vi "Linux ip route get.vi"(8 "error in (no error)":errorcluster, 11 "address":refnum<class "IPv4 Network Address.lvclass">) -> (0 "error out":errorcluster, 3 "ip route get stdout":string, 5 "ip route get stderr":string)   [LabVIEW 2020, in "NI_WFCN.lvlib" / "IPv4 Network Address.lvclass"]
doc: "Linux: call `ip route get $ip` to determine if the specified address is routable."
uses:
  <vilib>/net/WFCN/Addressing/IPv4 Network Address/IPv4 Network Address.lvclass
  <vilib>/net/WFCN/NI_WFCN.lvlib
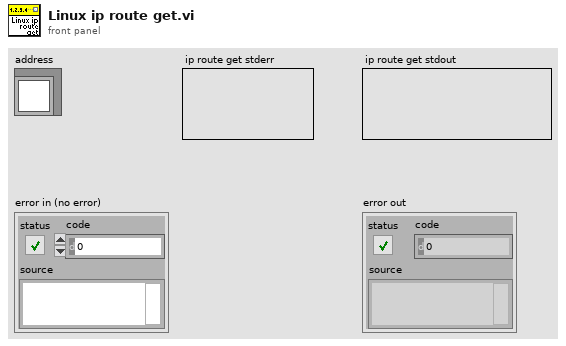
[diagram p1: front panel]
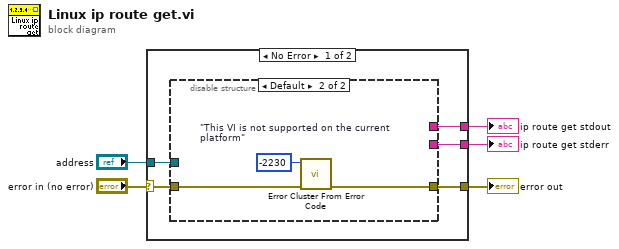
[diagram p0: block diagram]
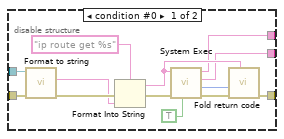
[diagram p2: hidden frame]
diagram:
  n1 = case shown="No Error" "error in (no error)" {
    selector: "error in (no error)" -> [w8 w27]
    tunnel: "address" -> [w10 _]
    tunnel: [w9 w27] -> w5
    tunnel: [w7 _] -> w2
    tunnel: [w6 _] -> w1
    frame No Error {
      n2 = disable-structure shown="Default" {
        disable-tunnel: w10 -> [w23 _]
        disable-tunnel: w8 -> [w22 w25]
        disable-tunnel: [w15 w24] -> w9
        disable-tunnel: [w12 _] -> w7
        disable-tunnel: [w11 _] -> w6
        frame condition #0 {
          n3 = call-dynamic "Format to string.vi"("error in (no error)"=w22, "address"=w23) -> ("error out"=w20:errorcluster, "address string"=w19:string)  [unwired: 7 in, 1 out]
          n4 = Format Into String(format string="ip route get %s", error in=w20, w19) -> (resulting string=w13:string, error out=w18:errorcluster)  [unwired: 1 in]
          n5 = call <vilib>:"System Exec.vi"("run minimized? (F)"=TRUE, "error in (no error)"=w18, "command line"=w13) -> ("error out"=w16:errorcluster, "return code"=w14:i32, "standard error"=w11:string, "standard output"=w12:string)  [unwired: 5 in]
          n6 = call <vilib>:"Fold return code.vi"("command"=w13, "error in (no error)"=w16, "return code"=w14) -> ("error out"=w15:errorcluster)  [unwired: 8 in]
        }
        frame condition #1 (active) {
          w26 = -2230  # "This VI is not supported on the current platform"
          n7 = call <vilib>:"Error Cluster From Error Code.vi"("error in (no error)"=w25, "error code (0)"=w26) -> ("error out"=w24:errorcluster)  [unwired: 7 in]
        }
      }
    }
    frame Error {
    }
  }
  "error out" <- w5
  "ip route get stdout" <- w2
  "ip route get stderr" <- w1
